vi "Event UI.vi"(8 "error in (no error)":errorcluster, 10 "Context In":refnum<class "ContextData.lvclass"> caption="Context DVR In", 11 "Wait Event in":refnum<class "Launch UI.lvclass">) -> (0 "error out":errorcluster, 3 "Wait Event out":refnum<class "Launch UI.lvclass">)   [LabVIEW 2020, in "Launch UI.lvclass"]
uses:
  Launch UI.lvclass
  UI Controls/redRoundButton.ctl
  ContextData/ContextData.lvclass
  State/State.lvclass
  Check Move/Check Move.lvclass
  C:/Users/fflores/Documents/GitHub Projects/Simon/Simon Game/OOP States/State/State.lvclass
  Check Move/Check Move.lvclass/Check Move.ctl
  Change Level/Change Level.lvclass
  Change Level/Change Level.lvclass/Change Level.ctl
  Start Game/Start Game.lvclass
  Start Game/Start Game.lvclass/Start Game.ctl
  Longest/Longest.lvclass
  Last/Last.lvclass
  Handle Menu Actions/Handle Menu Actions.lvclass
  Handle Menu Actions/Handle Menu Actions.lvclass/Handle Menu Actions.ctl
  Exit/Exit.lvclass
  Check Move/Accessors/setPressedButtonRef.vi
  Change Level/Accessors/setLevel.vi
  Start Game/Accessors/setUiViRefnum.vi
  Handle Menu Actions/Accessors/setMenuItemTag.vi
  Handle Menu Actions/Accessors/setUIMenuRef.vi
  Messages/simonMessages/simonMessages.lvclass
panel:
  in  "0008":bool caption="LAST"
  in  "0007":bool caption="LONGEST"
  in  "0006":T1 caption="START"
  in  "0005":u8(slide)=1 caption="LEVEL" min=1 max=5 step=1 scale=1.0..4.0
  in  "0001":bool caption="Red"
  in  "0004":bool caption="Yellow"
  in  "0003":bool caption="Green"
  in  "0002":bool caption="Blue"
  out "0009":string caption="DISPLAY"
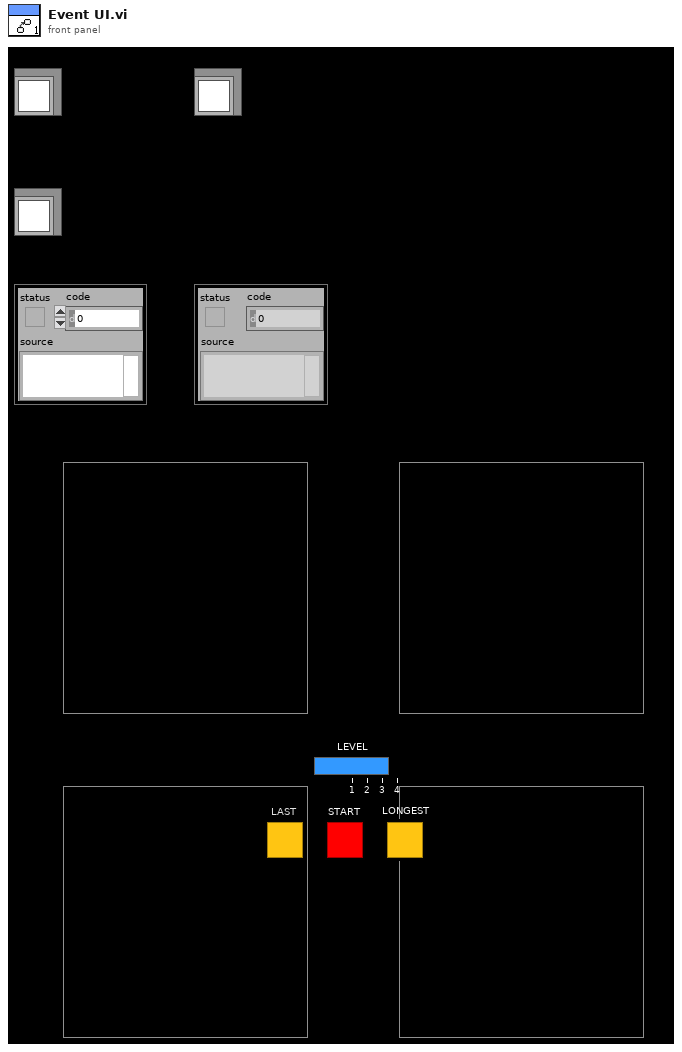
[diagram p1: front panel]
types:
  T1 = typedef "redRoundButton.ctl" = bool
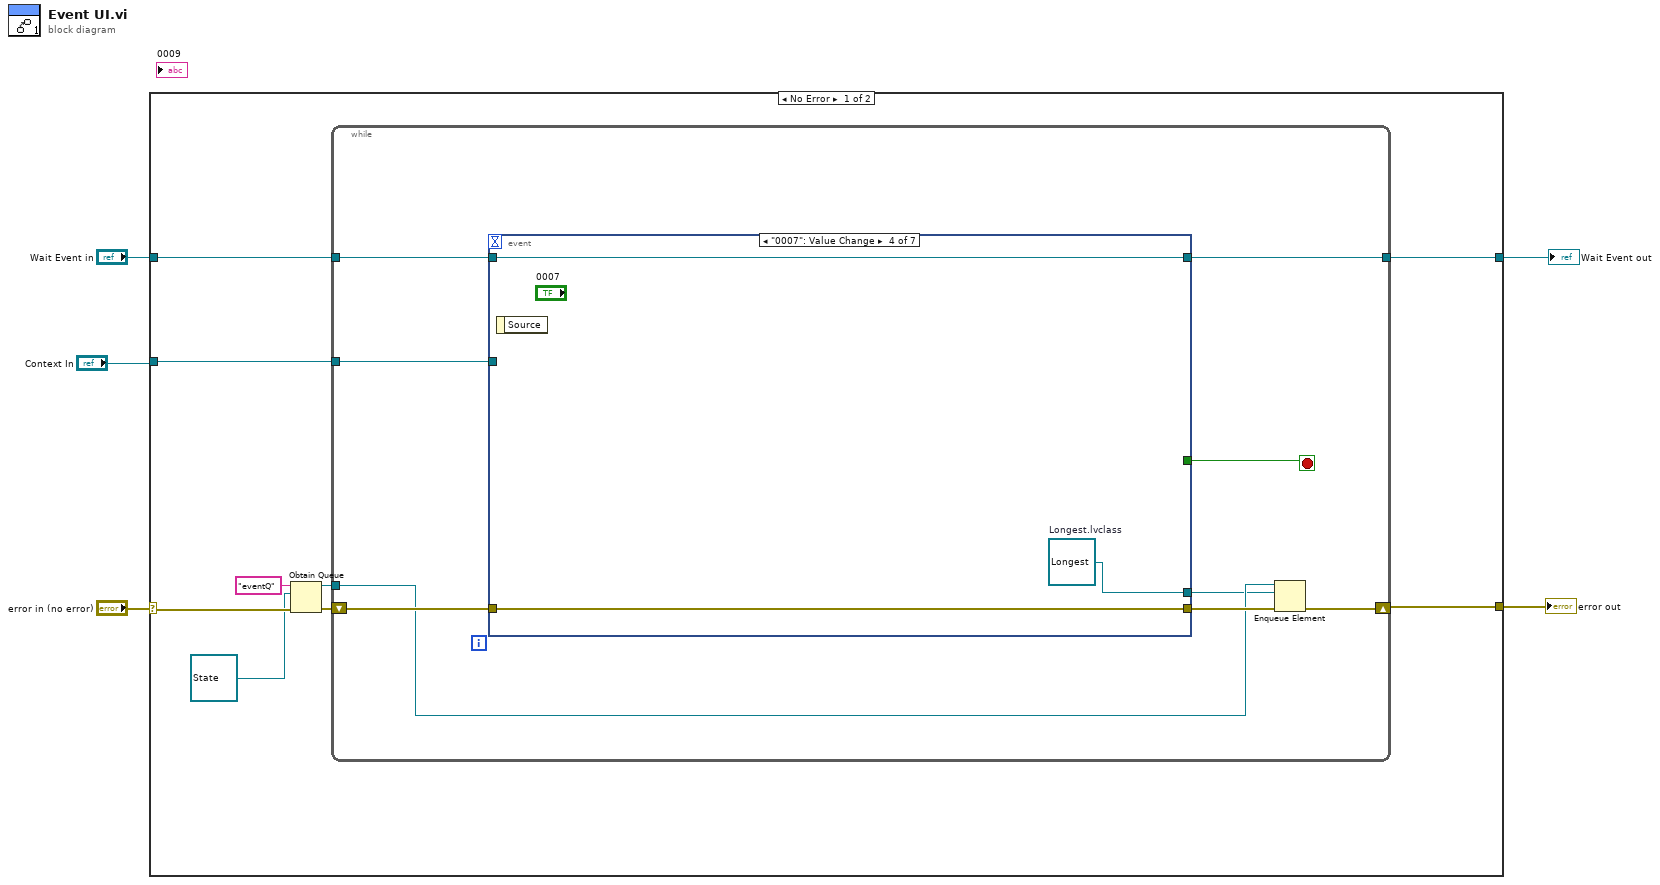
[diagram p0: block diagram]
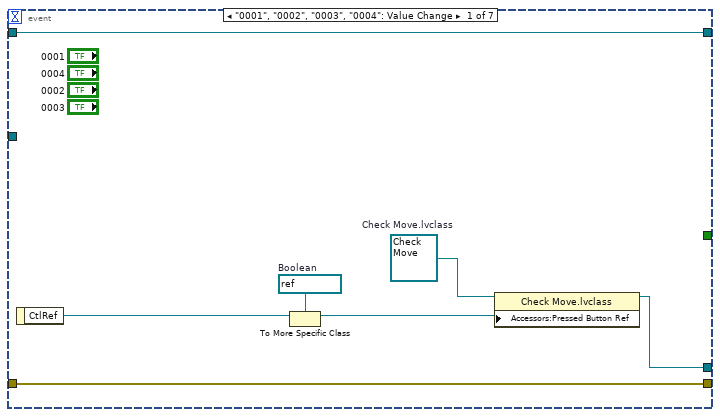
[diagram p2: hidden frame]
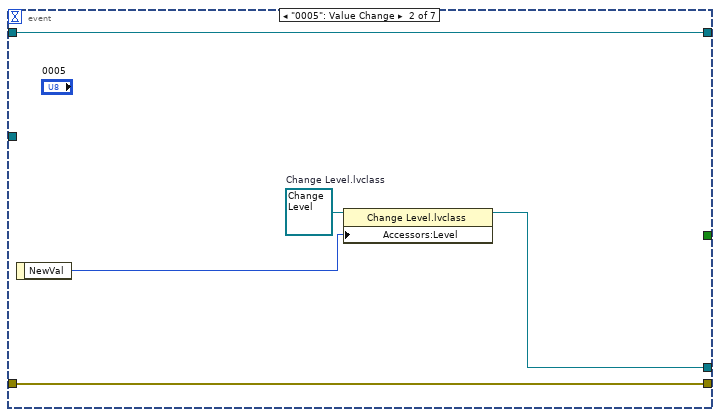
[diagram p3: hidden frame]
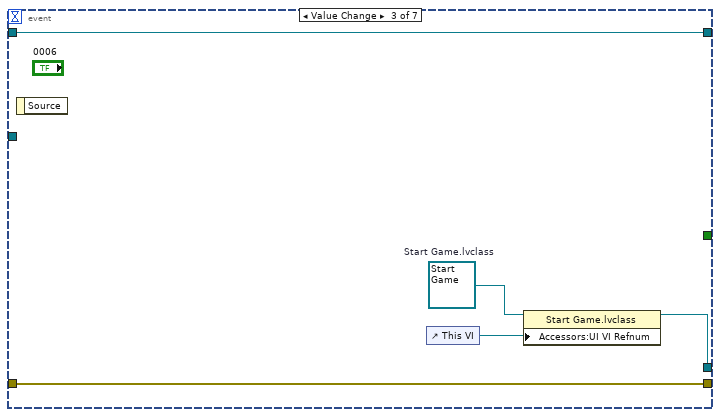
[diagram p4: hidden frame]
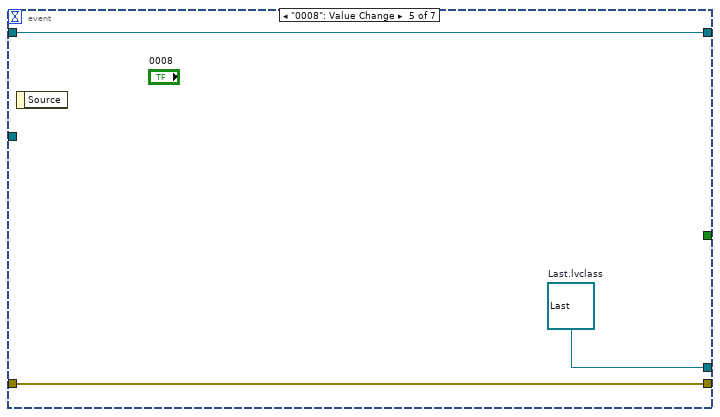
[diagram p5: hidden frame]
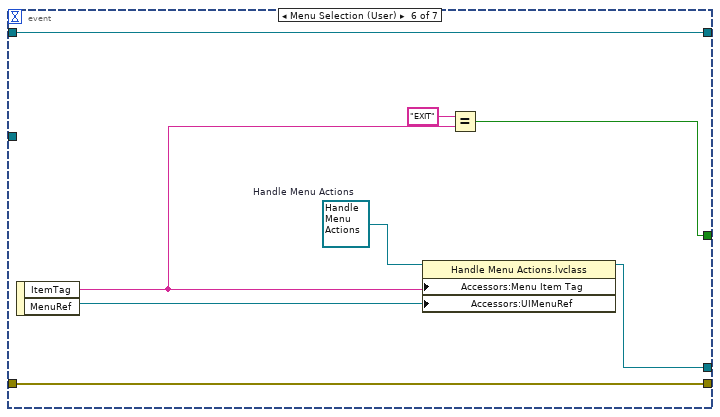
[diagram p6: hidden frame]
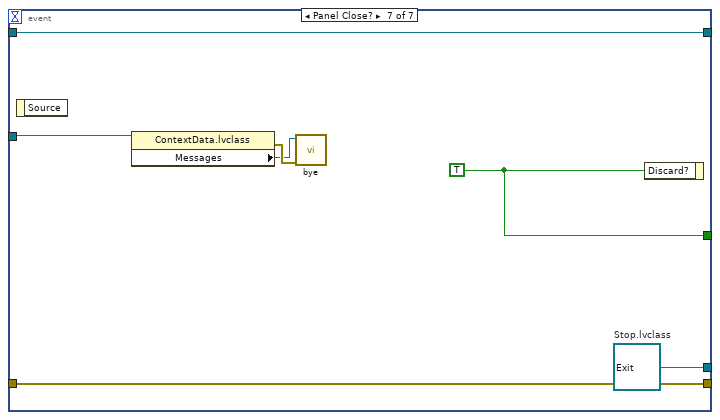
[diagram p7: hidden frame]
diagram:
  n1 = case shown="No Error" "error in (no error)" {
    selector: "error in (no error)" -> [w8 w63]
    tunnel: [w12 w63] -> w4
    tunnel: [w13 w62] -> w2
    tunnel: "Wait Event in" -> [w14 w62]
    tunnel: "Context In" -> [w11 _]
    frame No Error {
      n2 = Obtain Queue(name (unnamed)="eventQ", element data type=refnum<class "State.lvclass"> refnum ("Context DVR In"), error in (no error)=w8) -> (queue out=w7:refnum<queue>, error out=w9:errorcluster)  [unwired: 2 in, 1 out]
      n3 = while {
        tunnel: w14 -> [w23]
        tunnel: [w22] -> w13
        shift-right: [w18] -> w12
        shift-left: w9 -> [w21]
        tunnel: w11 -> [w19]
        tunnel: w7 -> [w17]
        stop <- w15 stop-if-true
        n4 = event shown="[3] \"0007\": Value Change" {
          selector: _ -> [_ _ _ _ _ _ _]
          dyn-events: _ -> [_ _ _ _ _ _ _]
          timeout: _ -> [_ _ _ _ _ _ _]
          tunnel: w23 -> [w30 w35 w40 w43 w46 w54 w61]
          tunnel: [w30 w35 w40 w43 w46 w54 w61] -> w22
          tunnel: w21 -> [w29 w33 w38 w42 w45 w53 w60]
          tunnel: [w29 w33 w38 w42 w45 w53 w60] -> w20
          tunnel: [_ _ _ _ _ w50 w58] -> w15
          tunnel: w19 -> [_ _ _ _ _ _ w56]
          tunnel: [w27 w32 w37 w41 w44 w51 w55] -> w16
          event "0001", "0002", "0003", "0004": Value Change {
            w24 = refnum<vi> refnum  # Boolean
            w28 = refnum<class "Check Move.lvclass"> refnum  # Check Move.lvclass
            n5 = event-data() -> ("CtlRef"=w26:refnum<vi>)  [unwired: 1 in]
            n6 = To More Specific Class(target class=w24, reference=w26) -> (specific class reference=w25:refnum<vi>)  [unwired: 1 in, 1 out]
            n7 = property class="Check Move.lvclass"(reference=w28, "Accessors:Pressed Button Ref"=w25) -> (reference out=w27:refnum<class "Check Move.lvclass">)  [unwired: 1 in, 1 out]
          }
          event "0005": Value Change {
            w34 = refnum<class "Change Level.lvclass"> refnum  # Change Level.lvclass
            n8 = event-data() -> ("NewVal"=w31:u8)  [unwired: 1 in]
            n9 = property class="Change Level.lvclass"(reference=w34, "Accessors:Level"=w31) -> (reference out=w32:refnum<class "Change Level.lvclass">)  [unwired: 1 in, 1 out]
          }
          event Value Change {
            w39 = refnum<class "Start Game.lvclass"> refnum  # Start Game.lvclass
            n10 = event-data() -> ()  [unwired: 1 in, 1 out]
            n11 = control-ref of="This VI"() -> (w36:refnum<vi>)
            n12 = property class="Start Game.lvclass"(reference=w39, "Accessors:UI VI Refnum"=w36) -> (reference out=w37:refnum<class "Start Game.lvclass">)  [unwired: 1 in, 1 out]
          }
          event "0007": Value Change {
            w41 = refnum<class "Longest.lvclass"> refnum  # Longest.lvclass
            n13 = event-data() -> ()  [unwired: 1 in, 1 out]
          }
          event "0008": Value Change {
            w44 = refnum<class "Last.lvclass"> refnum  # Last.lvclass
            n14 = event-data() -> ()  [unwired: 1 in, 1 out]
          }
          event Menu Selection (User) {
            w52 = refnum<class "Handle Menu Actions.lvclass"> refnum  # Handle Menu Actions
            n15 = event-data() -> ("ItemTag"=w49:string, "MenuRef"=w47:refnum<k9>)  [unwired: 1 in]
            n16 = property class="Handle Menu Actions.lvclass"(reference=w52, "Accessors:Menu Item Tag"=w49, "Accessors:UIMenuRef"=w47) -> (reference out=w51:refnum<class "Handle Menu Actions.lvclass">)  [unwired: 1 in, 1 out]
            n17 = Equal?(x="EXIT", y=w49) -> (x = y?=w50:bool)
          }
          event Panel Close? {
            w58 = TRUE ("Discard?")
            w55 = refnum<class "Exit.lvclass"> refnum  # Stop.lvclass
            n18 = event-data() -> ()  [unwired: 1 in, 1 out]
            n19 = property class="ContextData.lvclass"(reference=w56) -> (error out=w59:errorcluster, "Messages"=w57:refnum<class "simonMessages.lvclass">)  [unwired: 1 in, 1 out]
            n20 = call "bye.vi"("error in (no error)"=w59, "simonMessages in"=w57) -> ()  [unwired: 8 in, 2 out]
            n21 = event-data("Discard?"=w58) -> ()  [unwired: 1 in, 1 out]
          }
        }
        n22 = Enqueue Element(queue=w17, element=w16, error in (no error)=w20) -> (error out=w18:errorcluster)  [unwired: 1 in, 2 out]
      }
    }
    frame Error {
    }
  }
  "error out" <- w4
  "Wait Event out" <- w2
